vi "daq.io Get Device Events Example.vi"(8 "error in":errorcluster) -> (0 "error out":errorcluster)   [LabVIEW 2013, in "daqio minimal.lvlib"]
doc: "This example demonstrates how to read all Events that occured for a specific Device on daq.io."
uses:
  daqio minimal.lvlib
  _typedefs/update-button.ctl
  _typedefs/exmpl_overlay_mask.ctl
  _typedefs/daqio-Credentials.ctl
  _typedefs/daqio-Type.ctl
  <vilib>/httpClient/ClientHandle.ctl
  <vilib>/Platform/browser.llb/Open URL in Default Browser (string).vi
  <vilib>/httpClient/LabVIEWHTTPClient.lvlib
panel:
  out "overlay mask":T1
  out "Event View":string[][](table)
  in  "Retrieve Events":T2
  in  "Stop":bool
  out "connected to daq.io":bool
  in  "Sign up link":bool caption="Boolean"
  out "Device Key":string
  in  "Log On":bool
  in  "User Name (your email)":string
  in  "Password":string
  # "Get your free account at daq.io first: sign up at"
  # "This Machine"
  # "(autogenerated in this example)"
  # "Device Events"
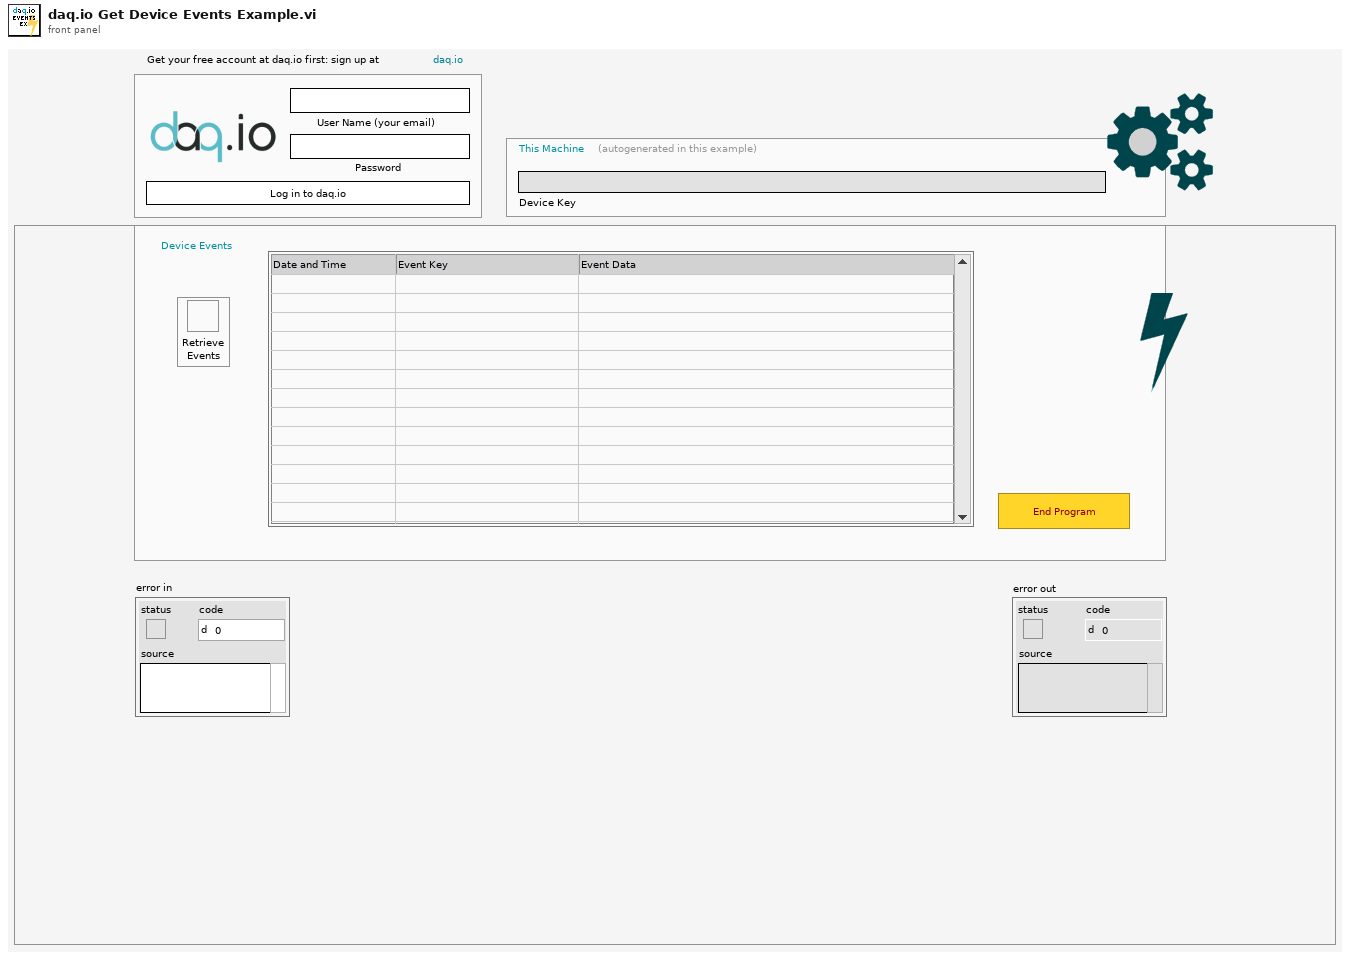
[diagram p1: front panel]
types:
  T1 = typedef "daqio minimal.lvlib/exmpl_overlay_mask.ctl" = bool
  T2 = typedef "daqio minimal.lvlib/update-button.ctl" = bool
  T3 = typedef "daqio minimal.lvlib/daqio-Credentials.ctl" = cluster{"User Name (email)":string, "Password":string}
  T4 = typedef "daqio minimal.lvlib/daqio-Type.ctl" = cluster{"daq.io ref":T5, "daq.io API Base":string, "Device Key":string, "Account ID":string, "online":bool, "SSL":bool, "buffer":bool}
  T5 = typedef "LabVIEWHTTPClient.lvlib/ClientHandle.ctl" = refnum<k1>
  T6 = cluster{"id":string, "key":string, "label":string}[]
  T7 = typedef "daqio minimal.lvlib/daqio-Event.ctl" = cluster{"device":string, "id":string, "value":string, "key":string, "time":string}
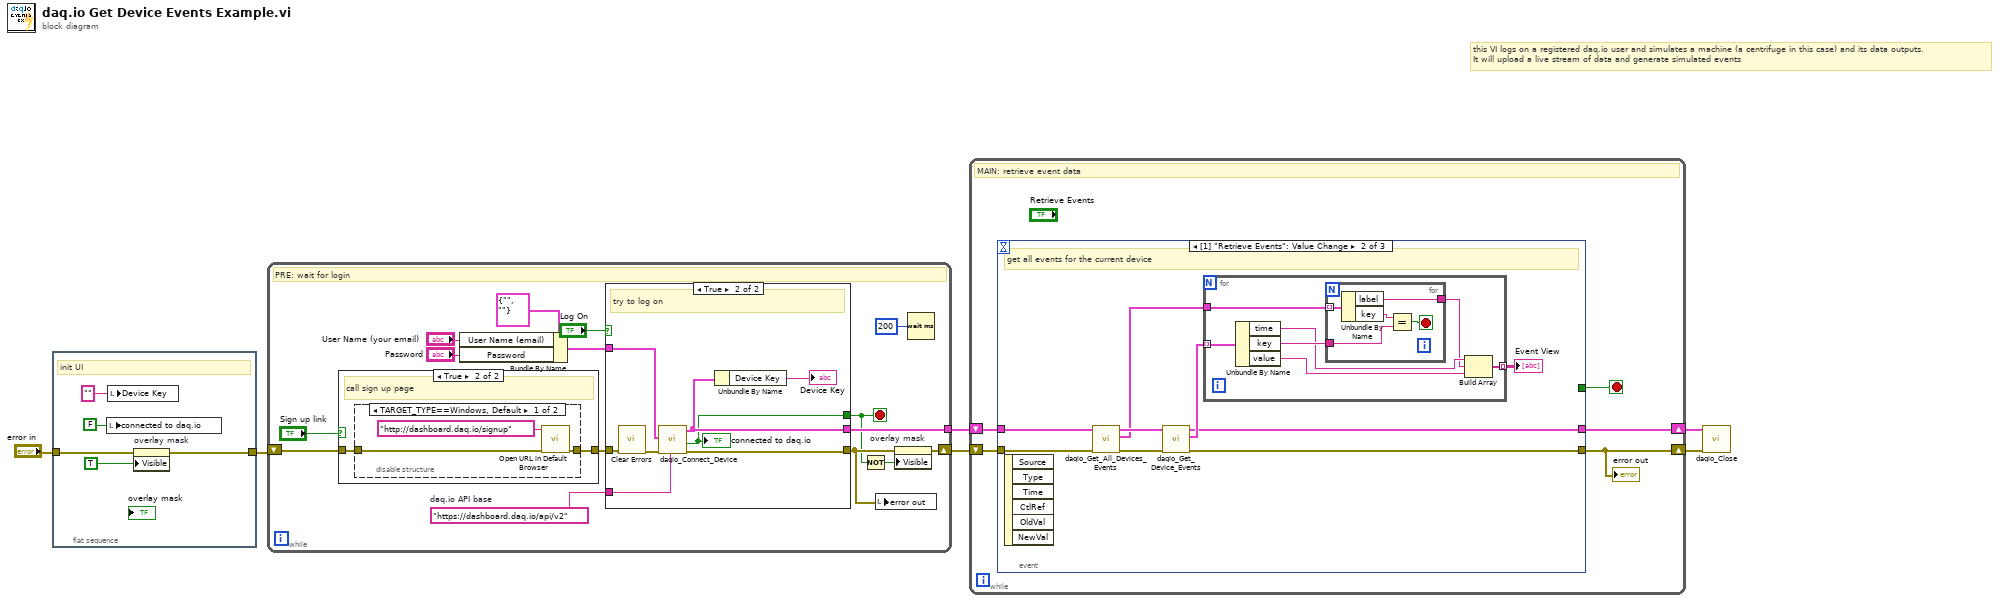
[diagram p0: block diagram]
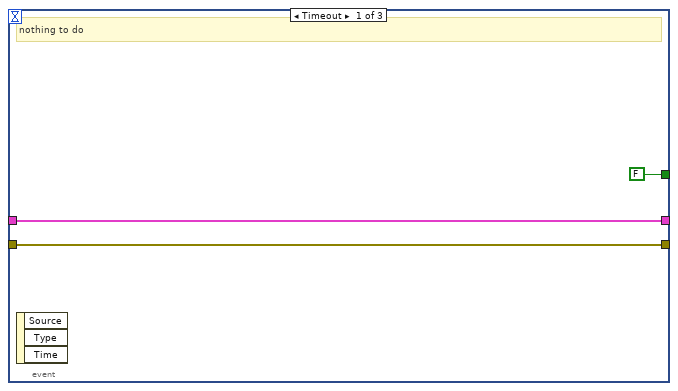
[diagram p2: hidden frame]
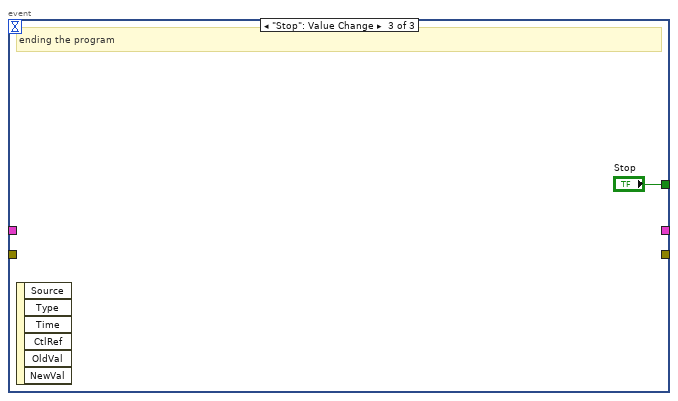
[diagram p3: hidden frame]
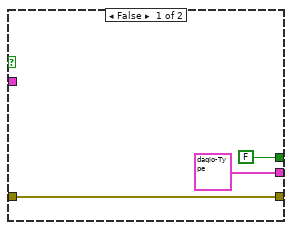
[diagram p6: hidden frame]
diagram:
  # "this VI logs on a registered daq.io user and simulates a machine (a centrifuge in this case) and its data outputs. \nIt will upload a live stream of data and generate simulated events"
  n1 = flat-sequence {
    tunnel: "error in" -> [w10]
    tunnel: [w9] -> w1
    frame #0 {
      # "init UI"
      n2 = local write "connected to daq.io"(FALSE ("connected to daq.io")) -> ()
      n3 = local write "Device Key"("" ("log")) -> ()
      n4 = property on="overlay mask" class="Bool (strict)"(error in=w10, "Visible"=TRUE) -> (error out=w9:errorcluster)  [unwired: 1 in, 1 out]
    }
  }
  n5 = while {
    shift-right: [w15] -> w3
    shift-left: w1 -> [w19]
    tunnel: [w21] -> w4
    stop <- w12 stop-if-true
    w16 = "https://dashboard.daq.io/api/v2"  # daq.io API base
    # "PRE: wait for login"
    n6 = case shown="True" "Sign up link" {
      tunnel: w19 -> [w27 w29]
      tunnel: [w27 w28] -> w18
      frame False {
      }
      frame True {
        # "call sign up page"
        n7 = disable-structure shown="TARGET_TYPE==Windows, Default" {
          disable-tunnel: w29 -> [w31 w33]
          disable-tunnel: [w30 w33] -> w28
          frame condition #0 (active) {
            n8 = call-poly <vilib>:"Open URL in Default Browser.vi"("error in (no error)"=w31, "URL"="http://dashboard.daq.io/signup") -> ("error out"=w30:errorcluster)  [unwired: 4 in, 1 out]
          }
          frame condition #1 {
          }
        }
      }
    }
    n9 = Bundle By Name(cluster=T3 {"User Name (email)"="", "Password"=""} ("daq.io Credentials"), "User Name (email)"="User Name (your email)", "Password"="Password") -> (w20:T3)
    n10 = case shown="True" "Log On" {
      tunnel: [T4 {"daq.io ref"=refnum, "daq.io API Base"="http://dashboard.daq.io/api/v1", "Device Key"="", "Account ID"="", "online"=FALSE, "SSL"=FALSE, "buffer"=FALSE} ("daq.io type out") w40] -> w21
      tunnel: [w34 w44] -> w14
      tunnel: w18 -> [w34 w43]
      tunnel: w16 -> [_ w42]
      tunnel: w20 -> [_ w41]
      tunnel: [FALSE ("connected successfully?") w38] -> w12
      frame False {
      }
      frame True {
        # "try to log on"
        n11 = call <vilib>:"Clear Errors.vi"("error in (no error)"=w43) -> ("error out"=w37:errorcluster)  [unwired: 6 in]
        n12 = call "daqio_Connect_Device.vi"("daq.io API base"=w42, "error in (no error)"=w37, "Credentials"=w41) -> ("error out"=w44:errorcluster, "connected successfully?"=w38:bool, "daq.io type out"=w40:T4)  [unwired: 6 in]
        "connected to daq.io" <- w38
        n13 = Unbundle By Name(w40) -> ("Device Key"=→"Device Key":string)
      }
    }
    n14 = Not(x=w12) -> (.not. x?=w13:bool)
    n15 = local write "error out"(w14) -> ()
    n16 = property on="overlay mask" class="Bool (strict)"(error in=w14, "Visible"=w13) -> (error out=w15:errorcluster)  [unwired: 1 in, 1 out]
    n17 = Wait (ms)(milliseconds to wait=u32 200) -> ()  [unwired: 1 out]
  }
  n18 = while {
    shift-right: [w45] -> w6
    shift-left: w3 -> [w48]
    shift-right: [w47] -> w2
    shift-left: w4 -> [w49]
    stop <- w46 stop-if-true
    # "MAIN: retrieve event data"
    n19 = event shown="[1] \"Retrieve Events\": Value Change" {
      selector: _ -> [_ _ _]
      dyn-events: _ -> [_ _ _]
      timeout: _ -> [_ _ _]
      tunnel: w49 -> [w51 w57 _]
      tunnel: w48 -> [w50 w56 _]
      tunnel: [w51 w59 _] -> w47
      tunnel: [w50 w58 _] -> w45
      tunnel: [FALSE ("Stop") _ "Stop"] -> w46
      event Timeout {
        # "nothing to do"
        n20 = event-data() -> ()  [unwired: 1 in, 3 out]
      }
      event Value Change {
        # "get all events for the current device"
        n21 = event-data() -> ()  [unwired: 1 in, 6 out]
        n22 = call "daqio_Get_All_Devices_Events.vi"("error in (no error)"=w56, "daq.io type in"=w57) -> ("error out"=w55:errorcluster, "All Device Events"=w53:T6, "daq.io type out"=w54:T4)  [unwired: 7 in]
        n23 = call "daqio_Get_Device_Events.vi"("error in (no error)"=w55, "daq.io type in"=w54) -> ("error out"=w58:errorcluster, "All Events"=w61:T7[], "daq.io type out"=w59:T4)  [unwired: 7 in]
        n24 = for {
          tunnel: w61 -> [w68] mode=indexing
          tunnel: [w63] -> w60 mode=indexing
          tunnel: w53 -> [w62]
          n25 = Unbundle By Name(w68) -> ("time"=w66:string, "key"=w67:string, "value"=w64:string)
          n26 = for {
            tunnel: w67 -> [w72]
            tunnel: [w70] -> w65
            tunnel: w62 -> [w69] mode=indexing
            stop <- w71 stop-if-true
            n27 = Unbundle By Name(w69) -> ("label"=w70:string, "key"=w73:string)
            n28 = Equal?(x=w73, y=w72) -> (x = y?=w71:bool)
          }
          n29 = Build Array(w66, w65, w64) -> (w63:string[])
        }
        "Event View" <- w60
      }
      event "Stop": Value Change {
        # "ending the program"
        n30 = event-data() -> ()  [unwired: 1 in, 6 out]
      }
    }
    "error out" <- w45
  }
  n31 = call "daqio_Close.vi"("error in (no error)"=w6, "daq.io type"=w2) -> ()  [unwired: 9 in, 1 out]
